vi "E3631A Power Supply.vi"(2 "error in (no error)":errorcluster, 4 "Data input":string) -> (0 "error out (no error)":errorcluster, 1 "Data output":string)   [LabVIEW 2011]
doc: "E3631A Power Supply\n\nHP E3631A Triple Output Power Supply VI, will set the voltage out put and current limit on the different channels.\n1: HPE3631A Channel 1 (0.0 - 6.18) V, (0.0 - 5.15) A\n2: HPE3631A Channel 2 (0.0 - 25.75) V, (0.0 - 1.03) A\n3: HPE3631A Channel 3 (-25.75 - 0.0) V, (0.0 - 1.03) A"
uses:
  <instrlib>/niDCPower/nidcpower.llb/niDCPower Sense.ctl
  <instrlib>/niDCPower/nidcpower.llb/niDCPower Output Function.ctl
  Server_Globals.vi
panel:
  in  "?":T1=1008 items=["Local"=1008, "Remote"=1009]
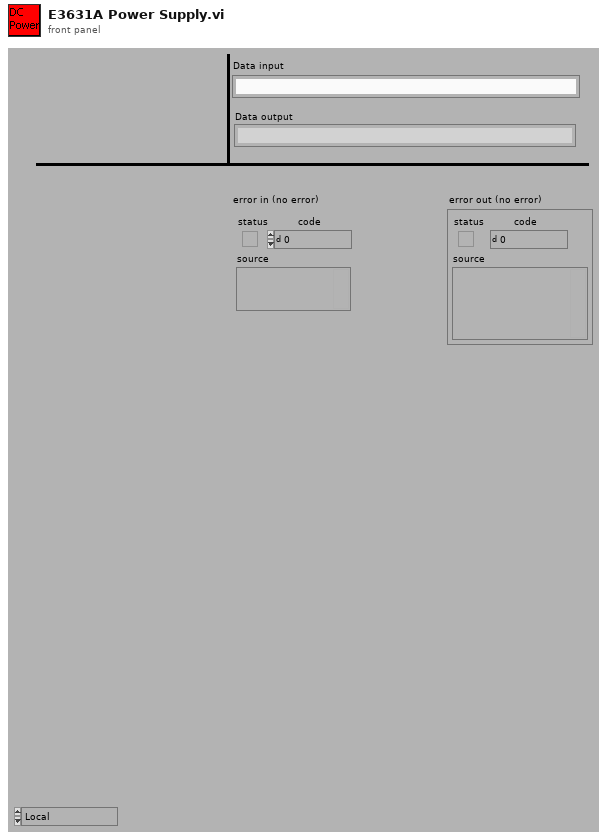
[diagram p1: front panel]
types:
  T1 = typedef "niDCPower Sense.ctl" = i32
  T2 = cluster{"I/O Settings":u64[], "Instrument Handle":cluster{"5402":refnum<k15>, " 5112":refnum<k15>, "4072":refnum<k15>, "USB":refnum<visa-resource-name>, "4110":refnum<k15>}, "Logfile":refnum<file>, "Log Level":i8, "Clear":i32[], "OS Set":cluster{"instrument handle out":refnum<k15>, "remaining string":string, "Settings":cluster{"Horizontal Conf.":cluster{"Min. Sample rate":dbl, "Reference position":dbl, "Record Length":i16}, "Channel A":cluster{"Enable":bool, "Vertical coupling":dbl, "Vertical range":dbl, "Vertical offset":dbl, "Probe attenuation":dbl}, "Channel B":cluster{"Enable":bool, "Vertical coupling":dbl, "Vertical range":dbl, "Vertical offset":dbl, "Probe attenuation":dbl}, "Trigger":cluster{"Source":enum8{"channel 1", "channel 2", "Imediate", "External trigger"}, "Slope":enum8{"Positive", "Negative"}, "Coupling":enum8{"AC", "DC"}, "Level":dbl, "Holdoff":dbl, "Delay":dbl, " Timeout":dbl, " Mode":enum8{"Normal", "Auto", "Auto Level"}}, "Measurements":cluster{"Measurement 1, Channel":enum8{"Channel 1", "Channel 2", "Channel 3", "Channel 4"}, "Measurement 1, Selection":u16, "Measurement 2, Channel":enum8{"Channel 1", "Channel 2", "Channel 3", "Channel 4"}, "Measurement 2,  Selection":u16, "Measurement 3, Channel":enum8{"Channel 1", "Channel 2", "Channel 3", "Channel 4"}, "Measurement 3, Selection 3":u16}}}, "DC Power Supply":cluster{"0":refnum<k15>, "1":refnum<k15>, "2":refnum<k15>, "3":refnum<k15>, "4":refnum<k15>}, "USB Interface":cluster{"0":refnum<visa-resource-name>, "1":refnum<visa-resource-name>, "2":refnum<visa-resource-name>, "3":refnum<visa-resource-name>, "4":refnum<visa-resource-name>}, "Function Generator":cluster{"0":refnum<k15>, "1":refnum<k15>, "2":refnum<k15>, "3":refnum<k15>, "4":refnum<k15>}, "Digital Multimeter":cluster{"0":refnum<k15>, "1":refnum<k15>, "2":refnum<k15>, "3":refnum<k15>, "4":refnum<k15>}, "Digital Osciliscope":cluster{"0":refnum<k15>, "1":refnum<k15>, "2":refnum<k15>, "3":refnum<k15>, "4":refnum<k15>}, "To M Server":string, "Adres":string[][], "Matrix version":string, "MD5":string, "Digital Multimeter Card 2":cluster{"0":string, "1":string, "2":string, "3":string, "4":string}}
  T3 = cluster{"0":refnum<k15>, "1":refnum<k15>, "2":refnum<k15>, "3":refnum<k15>, "4":refnum<k15>}
  T4 = typedef "niDCPower Output Function.ctl" = i32
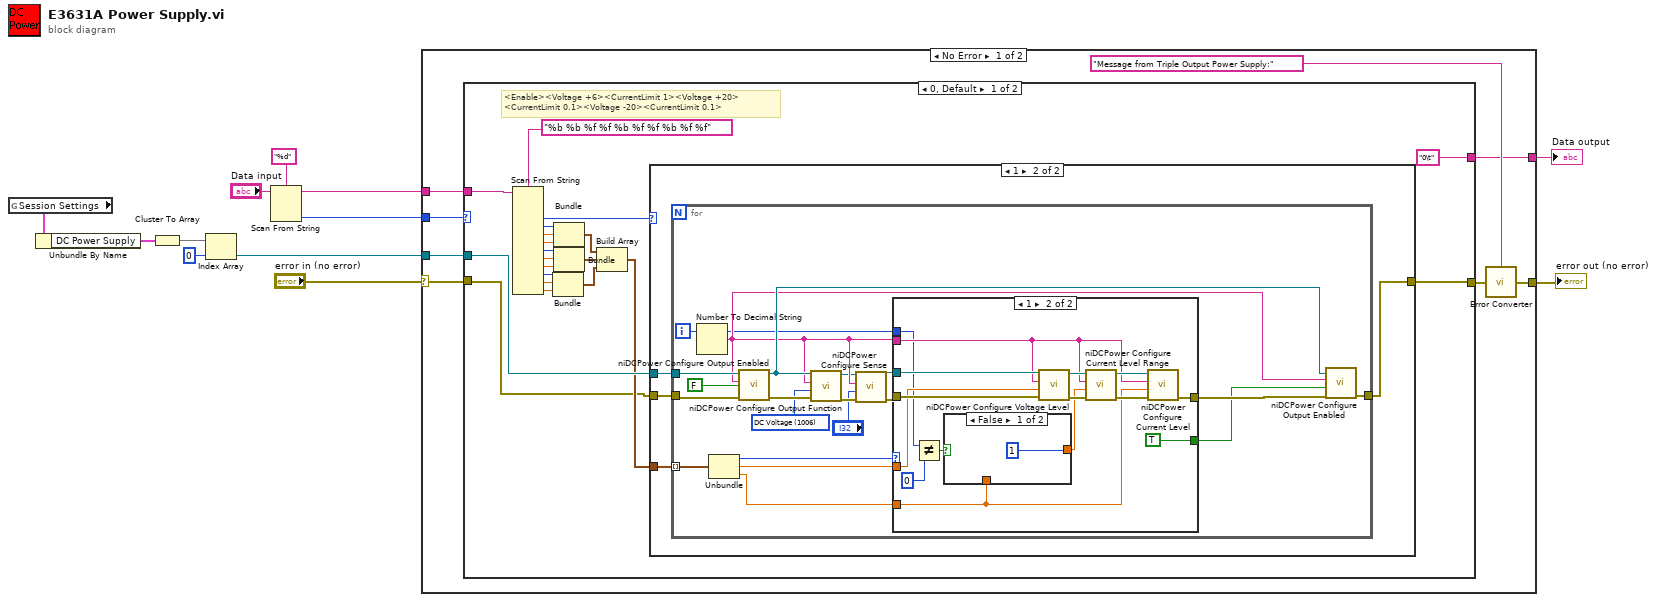
[diagram p0: block diagram]
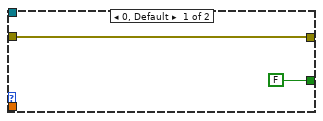
[diagram p3: hidden frame]
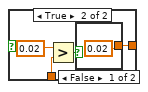
[diagram p4: hidden frame]
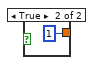
[diagram p5: hidden frame]
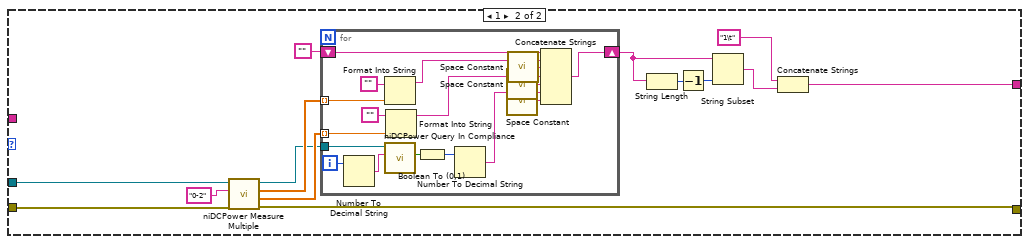
[diagram p6: hidden frame]
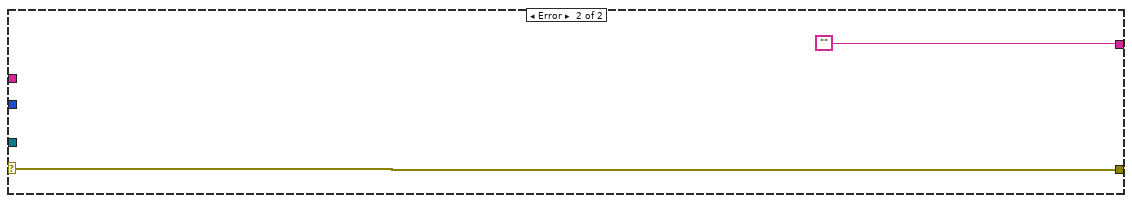
[diagram p7: hidden frame]
diagram:
  n1 = global read "Server_Globals.vi" "Session Settings"() -> (w7:T2)
  n2 = Unbundle By Name(w7) -> ("DC Power Supply"=w6:T3)
  n3 = Cluster To Array(cluster=w6) -> (array=w5:refnum<k15>[])
  n4 = Index Array(array=w5, index=0) -> (element=w3:refnum<k15>)
  n5 = Scan From String(format string="%d", input string="Data input") -> (remaining string=w2:string, output 1=w1:i32)  [unwired: 3 in, 2 out]
  n6 = case shown="No Error" "error in (no error)" {
    selector: "error in (no error)" -> [w17 w122]
    tunnel: [w19 w122] -> w12
    tunnel: w3 -> [w16 _]
    tunnel: [w15 ""] -> w10
    tunnel: w2 -> [w14 _]
    tunnel: w1 -> [w13 _]
    frame No Error {
      n7 = case shown="0, Default" w13 {
        tunnel: w17 -> [w21 w102]
        tunnel: [w40 w101] -> w18
        tunnel: w14 -> [w39 _]
        tunnel: w16 -> [w38 w94]
        tunnel: ["0\t" w93] -> w15
        frame 0, Default {
          # "<Enable><Voltage +6><CurrentLimit 1><Voltage +20>\n<CurrentLimit 0.1><Voltage -20><CurrentLimit 0.1>"
          n8 = Scan From String(format string="%b %b %f %f %b %f %f %b %f %f" ("Format String"), input string=w39) -> (output 1=w28:i32, output 2=w32:i32, output 3=w31:dbl, output 4=w30:dbl, output 5=w27:i32, output 6=w26:dbl, output 7=w25:dbl, output 8=w24:i32, output 9=w23:dbl, output 10=w22:dbl)  [unwired: 12 in, 3 out]
          n9 = Bundle(w24, w23, w22) -> (w33:cluster{i32, dbl, dbl})  [unwired: 1 in]
          n10 = Bundle(w32, w31, w30) -> (w35:cluster{i32, dbl, dbl})  [unwired: 1 in]
          n11 = Bundle(w27, w26, w25) -> (w34:cluster{i32, dbl, dbl})  [unwired: 1 in]
          n12 = Build Array(w35, w34, w33) -> (w29:cluster{i32, dbl, dbl}[])
          n13 = case shown="1" w28 {
            tunnel: w21 -> [w41 w45]
            tunnel: [w41 w44] -> w40
            tunnel: w38 -> [_ w43]
            tunnel: w29 -> [_ w42]
            frame 0, Default {
            }
            frame 1 {
              n14 = for {
                tunnel: w43 -> [w61]
                tunnel: w45 -> [w62]
                tunnel: [w64] -> w44
                tunnel: w42 -> [w59] mode=indexing
                i -> [w46]
                w52 = T4 1006 items=["DC Voltage"=1006, "DC Current"=1007] ("output function")
                n15 = Number To Decimal String(number=w46) -> (decimal integer string=w53:string)  [unwired: 1 in]
                n16 = Unbundle(w59) -> (w56:i32, w58:dbl, w57:dbl)
                n17 = call <instrlib>:"niDCPower Configure Output Enabled.vi"("error in (no error)"=w62, "output enabled"=FALSE, "channel name"=w53, "instrument handle"=w61) -> ("error out"=w63:errorcluster, "instrument handle out"=w54:refnum<k15>)  [unwired: 6 in]
                n18 = call <instrlib>:"niDCPower Configure Output Function.vi"("error in (no error)"=w63, "output function"=w52, "channel name"=w53, "instrument handle"=w54) -> ("error out"=w50:errorcluster, "instrument handle out"=w51:refnum<k15>)  [unwired: 6 in]
                n19 = call <instrlib>:"niDCPower Configure Sense.vi"("error in (no error)"=w50, "sense"="?", "channel name"=w53, "instrument handle"=w51) -> ("error out"=w49:errorcluster, "instrument handle out"=w47:refnum<k15>)  [unwired: 6 in]
                n20 = case shown="1" w56 {
                  tunnel: w47 -> [_ w78]
                  tunnel: w53 -> [_ w74]
                  tunnel: w58 -> [_ w73]
                  tunnel: w57 -> [_ w72]
                  tunnel: w49 -> [w67 w77]
                  tunnel: [w67 w82] -> w65
                  tunnel: [FALSE TRUE] -> w55
                  tunnel: w46 -> [_ w69]
                  frame 0, Default {
                  }
                  frame 1 {
                    n21 = Not Equal?(x=w69, y=0) -> (x != y?=w70:bool)
                    n22 = case shown="False" w70 {
                      tunnel: w72 -> [_ w86]
                      tunnel: [1 w84] -> w71
                      frame False {
                      }
                      frame True {
                        n23 = Greater?(x=0.02, y=w86) -> (0:w87:bool)
                        n24 = case shown="False" w87 {
                          tunnel: [0.02 1] -> w84
                          frame False {
                          }
                          frame True {
                          }
                        }
                      }
                    }
                    n25 = call <instrlib>:"niDCPower Configure Voltage Level.vi"("error in (no error)"=w77, "voltage level"=w73, "channel name"=w74, "instrument handle"=w78) -> ("error out"=w75:errorcluster, "instrument handle out"=w76:refnum<k15>)  [unwired: 6 in]
                    n26 = call <instrlib>:"niDCPower Configure Current Level Range.vi"("error in (no error)"=w75, "current level range"=w71, "channel name"=w74, "instrument handle"=w76) -> ("error out"=w79:errorcluster, "instrument handle out"=w80:refnum<k15>)  [unwired: 6 in]
                    n27 = call <instrlib>:"niDCPower Configure Current Level.vi"("error in (no error)"=w79, "current level"=w72, "channel name"=w74, "instrument handle"=w80) -> ("error out"=w82:errorcluster)  [unwired: 6 in, 1 out]
                  }
                }
                n28 = call <instrlib>:"niDCPower Configure Output Enabled.vi"("error in (no error)"=w65, "output enabled"=w55, "channel name"=w53, "instrument handle"=w54) -> ("error out"=w64:errorcluster)  [unwired: 6 in, 1 out]
              }
            }
          }
        }
        frame 1 {
          n29 = call <instrlib>:"niDCPower Measure Multiple.vi"("error in (no error)"=w102, "channel name"="0-2", "instrument handle"=w94) -> ("error out"=w101:errorcluster, "current measurements"=w99:dbl[], "voltage measurements"=w100:dbl[], "instrument handle out"=w90:refnum<k15>)  [unwired: 5 in]
          n30 = for {
            tunnel: w100 -> [w114] mode=indexing
            tunnel: w99 -> [w117] mode=indexing
            shift-right: [w120] -> w95
            shift-left: "" -> [w119]
            tunnel: w90 -> [w109]
            i -> [w108]
            n31 = Number To Decimal String(number=w108) -> (decimal integer string=w107:string)  [unwired: 1 in]
            n32 = Format Into String(initial string="", w114) -> (resulting string=w113:string)  [unwired: 2 in, 1 out]
            n33 = call <instrlib>:"niDCPower Query In Compliance.vi"("channel name"=w107, "instrument handle"=w109) -> ("in compliance?"=w106:bool)  [unwired: 7 in, 2 out]
            n34 = Format Into String(initial string="", w117) -> (resulting string=w116:string)  [unwired: 2 in, 1 out]
            n35 = Boolean To (0,1)(Boolean=w106) -> (0, 1=w105:i16)
            n36 = Number To Decimal String(number=w105) -> (decimal integer string=w104:string)  [unwired: 1 in]
            n37 = call <vilib>:"Space Constant.vi"() -> ("String"=w111:string)
            n38 = call <vilib>:"Space Constant.vi"() -> ("String"=w110:string)
            n39 = call <vilib>:"Space Constant.vi"() -> ("String"=w118:string)
            n40 = Concatenate Strings(w119, w113, w118, w116, w111, w104, w110) -> (w120:string)
          }
          n41 = String Length(string=w95) -> (length=w97:i32)
          n42 = Decrement(x=w97) -> (x-1=w96:i32)
          n43 = String Subset(string=w95, length (rest)=w96) -> (substring=w92:string)  [unwired: 1 in]
          n44 = Concatenate Strings("1\t", w92) -> (w93:string)
        }
      }
      n45 = call "Error Converter.vi"("error in (no error)"=w18, "String to add to error message"="Message from Triple Output Power Supply:" ("String to add message")) -> ("error out (no error)"=w19:errorcluster)
    }
    frame Error {
    }
  }
  "error out (no error)" <- w12
  "Data output" <- w10
